vi "Poll DMA.vi"(4 "Timeout is Error?":bool, 6 "Wait (ms)":u32=1, 8 "error in (no error)":errorcluster, 9 "Timeout (ms)":u32, 10 "Total Samples to Read":u32, 11 "Refs":T1={"Data Type"=enum."I32", "DMA_SGL"=refnum, "DMA_U64"=refnum, "DMA_I64"=refnum, "DMA_FXP+/-32.8"=refnum, "DMA_FXP+/-64.32"=refnum, "DMA_U32"=refnum, "DMA_U16"=refnum, "DMA_U8"=refnum, "DMA_I32"=refnum, "DMA_I16"=refnum, "DMA_I8"=refnum, "DMA_FXP+/-32.16"=refnum} {"Data Type" format="%.0x"}) -> (0 "error out":errorcluster, 3 "Refs":T1={"Data Type"=enum."I32", "DMA_SGL"=refnum, "DMA_U64"=refnum, "DMA_I64"=refnum, "DMA_FXP+/-32.8"=refnum, "DMA_FXP+/-64.32"=refnum, "DMA_U32"=refnum, "DMA_U16"=refnum, "DMA_U8"=refnum, "DMA_I32"=refnum, "DMA_I16"=refnum, "DMA_I8"=refnum, "DMA_FXP+/-32.16"=refnum} {"Data Type" format="%.0x"}, 5 "Timeout?":bool)   [LabVIEW 2017, in "FPGA Addon Engine.lvlib"]
uses:
  FPGA Addon Engine.lvlib
  Types/DMA Input Refs.ctl
  Shared/Data Type.ctl
  Shared/FPGA Addon Shared.lvlib
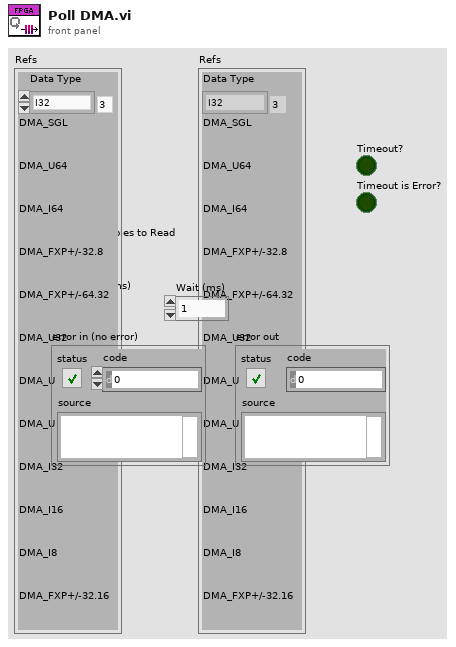
[diagram p1: front panel]
types:
  T1 = typedef "FPGA Addon Engine.lvlib/DMA Input Refs.ctl" = cluster{"Data Type":T2, "DMA_SGL":refnum<k20>, "DMA_U64":refnum<k20>, "DMA_I64":refnum<k20>, "DMA_FXP+/-32.8":refnum<k20>, "DMA_FXP+/-64.32":refnum<k20>, "DMA_U32":refnum<k20>, "DMA_U16":refnum<k20>, "DMA_U8":refnum<k20>, "DMA_I32":refnum<k20>, "DMA_I16":refnum<k20>, "DMA_I8":refnum<k20>, "DMA_FXP+/-32.16":refnum<k20>}
  T2 = typedef "FPGA Addon Shared.lvlib/Data Type.ctl" = enum8{"<Null>", "I8", "I16", "I32", "I64", "U8", "U16", "U32", "U64", "SGL", "Boolean", "Analog PWM In Settings", "Analog PWM In", "Digital PWM In Settings", "Digital PWM In", "Digital PWM Out", "Sine Out", "FXP+/-24.5", "FXP+/-16.5", "FXP+/-32.8", "FXP+/-64.32", "FXP+/-16.7", "FXP+/-20.5", "FXP+/-27.5", "FXP+/-32.16", "Digital Static In", "Digital Static Out", "Digital Static In Settings", "Digital WSS Out"}
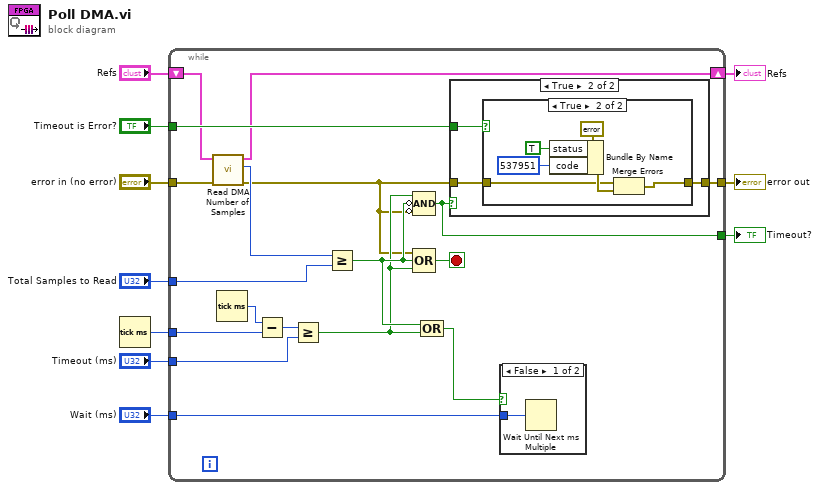
[diagram p0: block diagram]
diagram:
  n1 = Tick Count (ms)() -> (millisecond timer value=w10:u32)
  n2 = while {
    tunnel: "error in (no error)" -> [w11]
    tunnel: w10 -> [w27]
    tunnel: "Timeout (ms)" -> [w26]
    tunnel: [w25] -> w7
    tunnel: "Total Samples to Read" -> [w24]
    tunnel: "Wait (ms)" -> [w23]
    tunnel: [w21] -> w2
    tunnel: "Timeout is Error?" -> [w20]
    shift-right: [w12] -> w8
    shift-left: "Refs" -> [w13]
    stop <- w19 stop-if-true
    n3 = call "Read DMA Number of Samples.vi"("error in (no error)"=w11, "Refs in"=w13) -> ("error out"=w14:errorcluster, "Elements Remaining"=w15:u32, "Refs out"=w12:T1)  [unwired: 7 in]
    n4 = Tick Count (ms)() -> (millisecond timer value=w28:u32)
    n5 = Subtract(x=w28, y=w27) -> (x-y=w22:u32)
    n6 = Greater Or Equal?(x=w22, y=w26) -> (x >= y?=w17:bool)
    n7 = Greater Or Equal?(x=w15, y=w24) -> (x >= y?=w18:bool)
    n8 = Compound Arithmetic op=AND(w17, invert w18, invert w14) -> (w21:bool)
    n9 = Compound Arithmetic op=OR(w14, w18, w17) -> (w19:bool)
    n10 = Compound Arithmetic op=OR(w18, w17) -> (w16:bool)
    n11 = case shown="True" w21 {
      tunnel: w14 -> [w30 w33]
      tunnel: [w30 w32] -> w25
      tunnel: w20 -> [_ w31]
      frame False {
      }
      frame True {
        n12 = case shown="True" w31 {
          tunnel: w33 -> [w34 w37]
          tunnel: [w34 w36] -> w32
          frame False {
          }
          frame True {
            n13 = Bundle By Name(cluster=errorcluster {"status"=FALSE, "code"=0, "source"=""} ("error constant"), "status"=TRUE, "code"=537951) -> (w39:errorcluster)
            n14 = Merge Errors(w37, w39) -> (w36:errorcluster)
          }
        }
      }
    }
    n15 = case shown="False" w16 {
      tunnel: w23 -> [w29 _]
      frame False {
        n16 = Wait Until Next ms Multiple(millisecond multiple=w29) -> ()  [unwired: 1 out]
      }
      frame True {
      }
    }
  }
  "Refs" <- w8
  "error out" <- w7
  "Timeout?" <- w2
